vi "XYZ_translation_LastVersion.vi"() -> ()   [LabVIEW 2021]
uses:
  C:/Program Files (x86)/Control/SC3U.dll
  Program Files (x86)/Control/SC3U.dll
  <instrlib>/Xbox-One-Controller/Private/Type Defs/Indicators/Controller.ctl
  <instrlib>/Xbox-One-Controller/Private/Type Defs/Indicators/A.ctl
  <instrlib>/Xbox-One-Controller/Private/Type Defs/Indicators/B.ctl
  <instrlib>/Xbox-One-Controller/Private/Type Defs/Indicators/X.ctl
  <instrlib>/Xbox-One-Controller/Private/Type Defs/Indicators/Y.ctl
  <instrlib>/Xbox-One-Controller/Private/Type Defs/Indicators/Left Bumper.ctl
  <instrlib>/Xbox-One-Controller/Private/Type Defs/Indicators/Right Bumper.ctl
  <instrlib>/Xbox-One-Controller/Private/Type Defs/Indicators/View.ctl
  <instrlib>/Xbox-One-Controller/Private/Type Defs/Indicators/Menu.ctl
  <instrlib>/Xbox-One-Controller/Private/Type Defs/Indicators/Thumbstick_Analog.ctl
  <instrlib>/Xbox-One-Controller/Private/Type Defs/Indicators/Slider.ctl
  <instrlib>/Xbox-One-Controller/Private/Type Defs/Indicators/DPad.ctl
  <vilib>/Platform/TimedLoop/XDataNode/timing_clust.ctl
  <vilib>/Platform/TimedLoop/XDataNode/nitl_modes.ctl
  <vilib>/Platform/TimedLoop/XDataNode/wakeup.ctl
  <instrlib>/Xbox-One-Controller/Public/Open First Controller.vi
  <vilib>/Platform/TimedLoop/XDataNode/XDataNode.xnode
  <vilib>/Platform/TimedLoop/XDataNode/XDNodeRunTimeDep.lvlib
  <instrlib>/Xbox-One-Controller/LMH-Xbox-One-Controller.lvlib
panel:
  in  "Front Panel Window:Is Frontmost":bool
  in  "Displace Divided by 5":bool caption="Boolean 2"
  in  "Displace Multip by 5":bool caption="Boolean"
  out "Pos X":dbl
  out "Pos Z":dbl
  in  "Com Close 3":bool
  in  "Displace Z":i64=1
  out "Pos Y mm":dbl
  in  "Displace Y":i64
  in  "Com Close 2":bool
  in  "Stop Button":bool
  out "Controller":T1={"A Button"=FALSE, "B Button"=FALSE, "X Button"=FALSE, "Y Button"=FALSE, "Left Bumper"=FALSE, "Right Bumper"=FALSE, "View Button"=FALSE, "Menu Button"=FALSE, "Left Stick"={[], []}, "Right Stick"={[], []}, "Trigger"=0, "D-Pad"=5} {"Trigger" scale=32767.0..-32768.0}
  in  "SC3U":refnum<k24>(container)
  in  "Com Close":bool
  in  "Displace X":i64
  out "ConnectStatus":bool
  out "ComUsing":i16
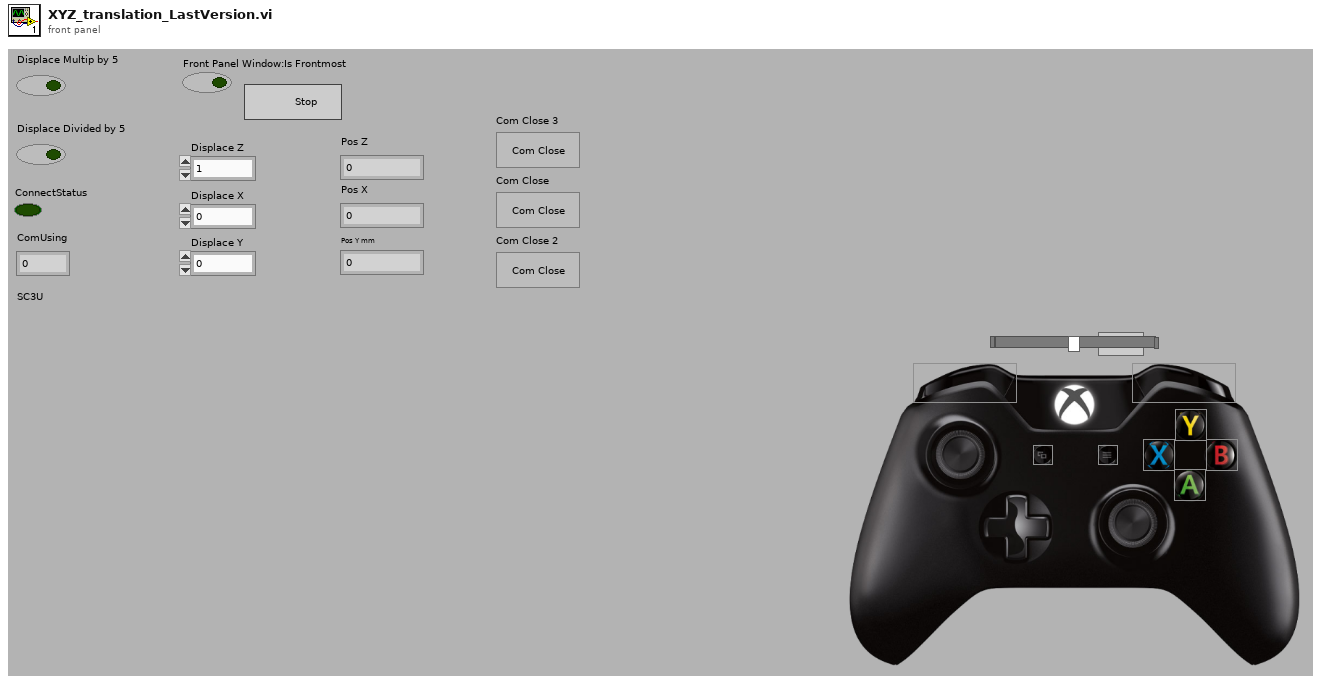
[diagram p1: front panel]
types:
  T1 = typedef "LMH-Xbox-One-Controller.lvlib/Controller.ctl" = cluster{"A Button":T2, "B Button":T3, "X Button":T4, "Y Button":T5, "Left Bumper":T6, "Right Bumper":T7, "View Button":T8, "Menu Button":T9, "Left Stick":T10, "Right Stick":T10, "Trigger":T11, "D-Pad":T12}
  T2 = typedef "LMH-Xbox-One-Controller.lvlib/A.ctl" = bool
  T3 = typedef "LMH-Xbox-One-Controller.lvlib/B.ctl" = bool
  T4 = typedef "LMH-Xbox-One-Controller.lvlib/X.ctl" = bool
  T5 = typedef "LMH-Xbox-One-Controller.lvlib/Y.ctl" = bool
  T6 = typedef "LMH-Xbox-One-Controller.lvlib/Left Bumper.ctl" = bool
  T7 = typedef "LMH-Xbox-One-Controller.lvlib/Right Bumper.ctl" = bool
  T8 = typedef "LMH-Xbox-One-Controller.lvlib/View.ctl" = bool
  T9 = typedef "LMH-Xbox-One-Controller.lvlib/Menu.ctl" = bool
  T10 = typedef "LMH-Xbox-One-Controller.lvlib/Thumbstick_Analog.ctl" = cluster{i32[], i32[]}
  T11 = typedef "LMH-Xbox-One-Controller.lvlib/Slider.ctl" = i32
  T12 = typedef "LMH-Xbox-One-Controller.lvlib/DPad.ctl" = u16
  T13 = typedef "XDNodeRunTimeDep.lvlib/timing_clust.ctl" = cluster{"Expected End [f-1]":u64, "Actual End [f-1]":u64, "Finished Late? [f-1]":bool, "Expected End [i-1]":u64, "Actual End [i-1]":u64, "Finished Late? [i-1]":bool, "Expected Start [i]":u64, "Actual Start [i]":u64, "Expected Start [f]":u64, "Actual Start [f]":u64, "Source Name":string, "Structure Name":string, "Period":i64, "Deadline":i64, "Offset":i64, "Start":i64, "Priority":i32, "Timeout":i32, "Mode":T14, "Wakeup Reason":T15, "Error":errorcluster, "Source Type":string, "Secondary Source Type":string, "Global End Time":u64, "Global Start Time":u64, "Frame Duration":u64, "Iteration Duration":u64, "Assigned CPU":i32, "I/O Scan Engine Mode":u32}
  T14 = typedef "XDNodeRunTimeDep.lvlib/nitl_modes.ctl" = enum32{"No Change", "Process missed periods, maintain original phase", "Discard missed periods, maintain original phase", "Process missed periods, ignore original phase", "Discard missed periods, ignore original phase"}
  T15 = typedef "XDNodeRunTimeDep.lvlib/wakeup.ctl" = enum32{"Normal", "Aborted", "Asynchronous wakeup", "Timing source error", "Timed loop error", "Timeout"}
  T16 = typedef "LMH-Xbox-One-Controller.lvlib/Xbox One Controller Ref.ctl" = cluster{"Controller Ref":refnum<k1>, "Event Refnum":refnum<event-registration>, "Worker Ref":refnum<vi>}
  T17 = typedef "LMH-Xbox-One-Controller.lvlib/All Axis Data.ctl" = cluster{"Left Stick":cluster{"X Axis":i32, "Y Axis":i32}, "Right Stick":cluster{"X Axis":i32, "Y Axis":i32}, "Triggers":i32, "D-Pad":T18}
  T18 = typedef "LMH-Xbox-One-Controller.lvlib/DPad Enum.ctl" = enum16{"Idle", "Up", "Up / Right", "Right", "Down / Right", "Down", "Down / Left", "Left", "Up / Left"}
  T19 = typedef "LMH-Xbox-One-Controller.lvlib/All Buttons Visual.ctl" = cluster{"A":T2, "B":T3, "X":T4, "Y":T5, "Left Bumper":T6, "Right Bumper":T7, "View Button":T8, "Menu Button":T9, "Left Stick":T20, "Right Stick":T20}
  T20 = typedef "LMH-Xbox-One-Controller.lvlib/Thumbstick.ctl" = bool
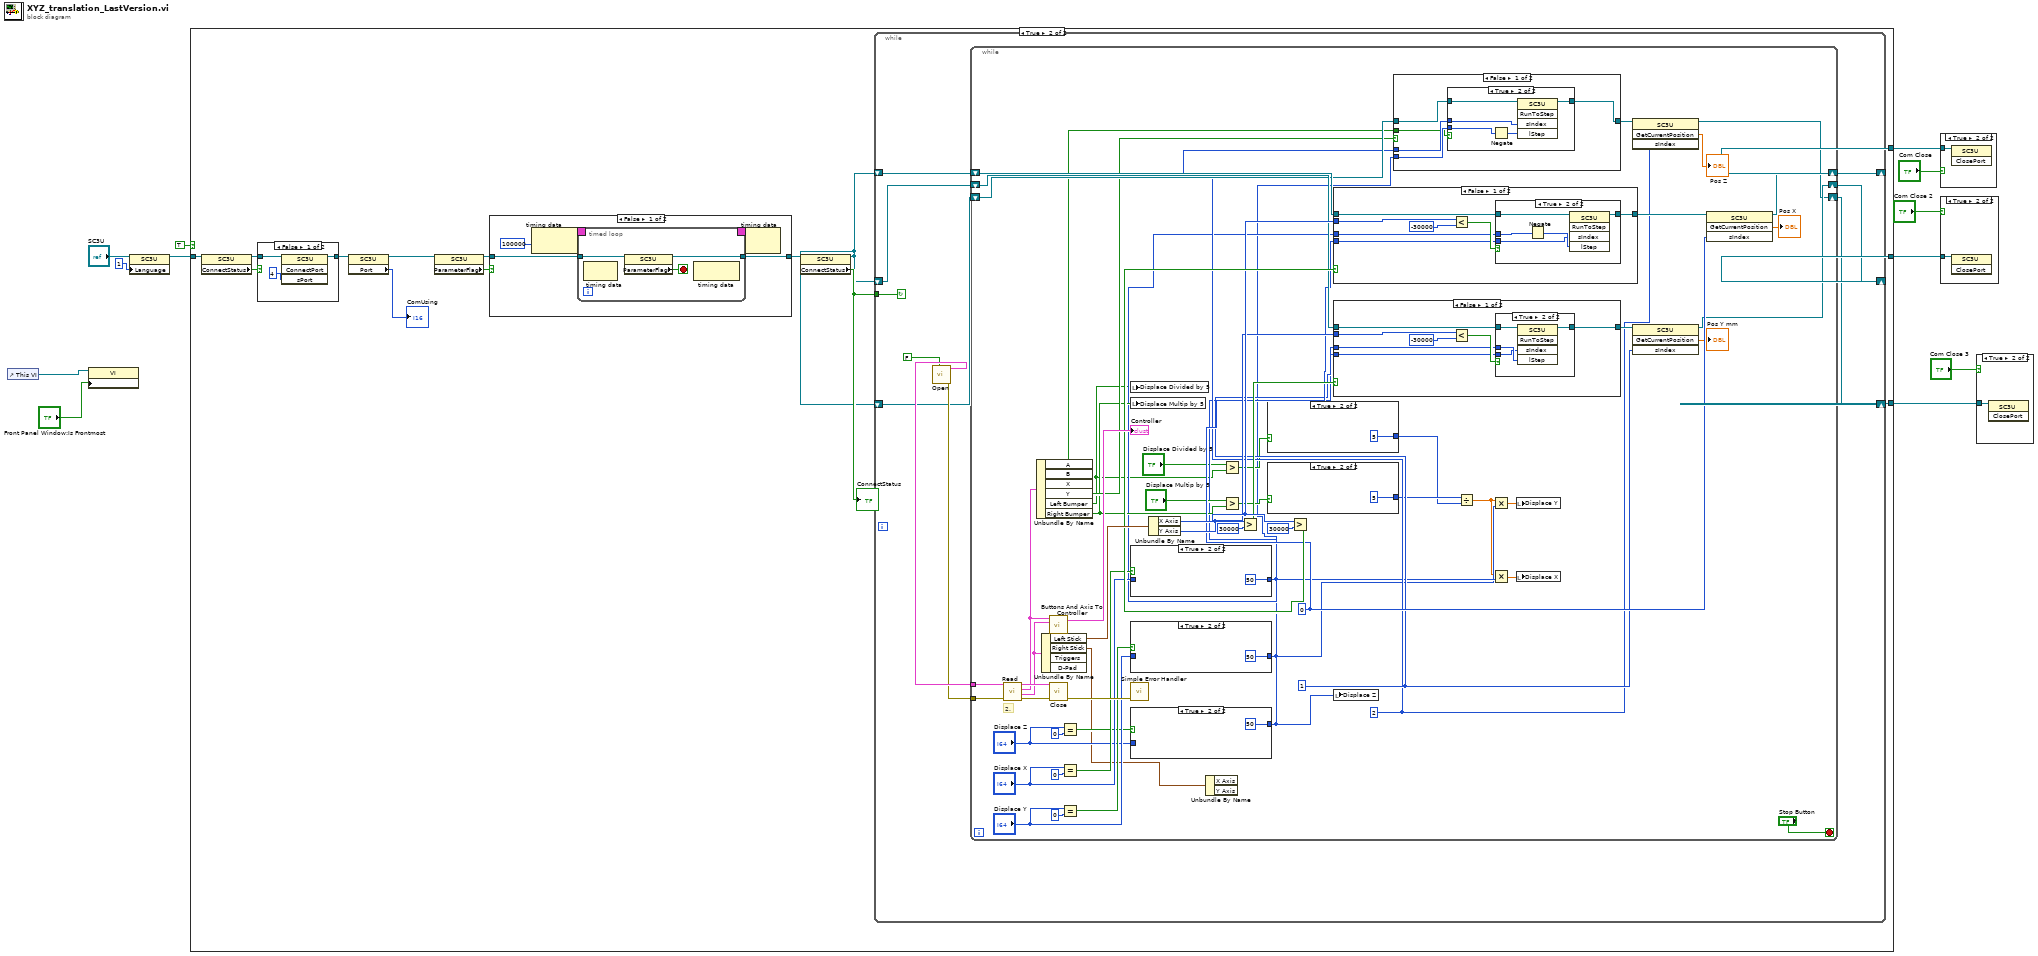
[diagram p0: block diagram]
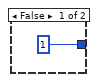
[diagram p7: hidden frame]
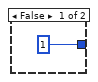
[diagram p9: hidden frame]
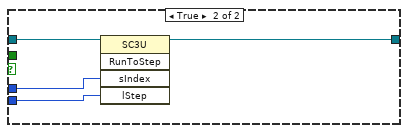
[diagram p12: hidden frame]
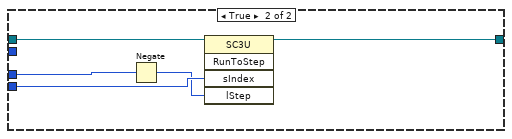
[diagram p14: hidden frame]
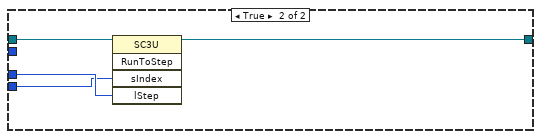
[diagram p16: hidden frame]
diagram:
  n1 = control-ref of="This VI"() -> (w2:refnum<vi>)
  n2 = property class="VI"(reference=w2, "Front Panel.IsFrontmost"="Front Panel Window:Is Frontmost") -> ()  [unwired: 1 in, 2 out]
  n3 = property class="SC3U"(reference="SC3U", "Language"=i16 1 ("intLanguage")) -> (reference out=w5:refnum<k24>)  [unwired: 1 in, 1 out]
  n4 = case shown="True" TRUE {
    tunnel: [_ w16] -> w8
    tunnel: w5 -> [_ w25]
    tunnel: [_ w15] -> w6
    tunnel: [_ w13] -> w3
    frame False {
    }
    frame True {
      n5 = property class="SC3U"(reference=w25) -> (reference out=w24:refnum<k24>, "ConnectStatus"=w23:bool)  [unwired: 1 in, 1 out]
      n6 = case shown="False" w23 {
        tunnel: w24 -> [w170 w171]
        tunnel: [w169 w171] -> w22
        frame False {
          n7 = invoke class="SC3U" method="ConnectPort"(reference=w170, "sPort"=i16 4 ("ComUsing")) -> (reference out=w169:refnum<k24>)  [unwired: 2 in, 3 out]
        }
        frame True {
        }
      }
      n8 = property class="SC3U"(reference=w22) -> (reference out=w20:refnum<k24>, "Port"=→"ComUsing":i16)  [unwired: 1 in, 1 out]
      n9 = property class="SC3U"(reference=w20) -> (reference out=w19:refnum<k24>, "ParameterFlag"=w18:bool)  [unwired: 1 in, 1 out]
      n10 = case shown="False" w18 {
        tunnel: w19 -> [w154 w167]
        tunnel: [w153 w167] -> w26
        frame False {
          n11 = node-c288(i64 100000 ("周期")) -> (w157:T13)
          n12 = timed-loop {
            timing: w157 -> [_]
            timing-out: [_] -> w156
            tunnel: w154 -> [w160]
            tunnel: [w159] -> w153
            stop <- w158 stop-if-true
            n13 = node-c288() -> ()  [unwired: 1 in, 1 out]
            n14 = property class="SC3U"(reference=w160) -> (reference out=w159:refnum<k24>, "ParameterFlag"=w158:bool)  [unwired: 1 in, 1 out]
            n15 = node-c288() -> ()  [unwired: 1 in, 1 out]
          }
          n16 = node-c288(w156) -> ()  [unwired: 1 out]
        }
        frame True {
        }
      }
      n17 = property class="SC3U"(reference=w26) -> (reference out=w14:refnum<k24>, "ConnectStatus"=w17:bool)  [unwired: 1 in, 1 out]
      "ConnectStatus" <- w17
      n18 = while {
        shift-right: [w36] -> w16
        shift-left: w14 -> [w35]
        tunnel: w17 -> [w34]
        shift-right: [w29] -> w15
        shift-left: w14 -> [w30]
        shift-right: [w27] -> w13
        shift-left: w14 -> [w28]
        stop <- w34 continue-if-true
        n19 = call-poly <instrlib>:"Open.vi"("Enable Events (T)"=FALSE) -> ("Error Out"=w32:errorcluster, "Xbox One Controller"=w33:T16)  [unwired: 8 in, 1 out]
        n20 = while {
          tunnel: w33 -> [w90]
          tunnel: w32 -> [w89]
          shift-right: [w76] -> w36
          shift-left: w35 -> [w93]
          shift-right: [w73] -> w29
          shift-left: w30 -> [w79]
          shift-right: [w67] -> w27
          shift-left: w28 -> [w68]
          stop <- "Stop Button" stop-if-true
          w66 = 2
          w71 = 1
          w75 = 0
          # "2."
          n21 = call <instrlib>:"Read.vi"("Error In"=w89, "Xbox One Controller Ref"=w90) -> ("Error Out"=w87:errorcluster, "All Axis"=w85:T17, "Buttons"=w64:T19, "Xbox One Controller Ref"=w86:T16)  [unwired: 6 in]
          n22 = Unbundle By Name(w64) -> ("A"=w63:T2, "Y"=w62:T5, "Left Bumper"=w46:T6, "Right Bumper"=w57:T7)  [unwired: 2 out]
          n23 = Unbundle By Name(w85) -> ("Left Stick"=w92:cluster{"X Axis":i32, "Y Axis":i32}, "Right Stick"=w37:cluster{"X Axis":i32, "Y Axis":i32})  [unwired: 2 out]
          n24 = call <instrlib>:"Buttons And Axis To Controller.vi"("All Axis"=w85, "Buttons"=w64) -> ("Controller"=→"Controller":T1)  [unwired: 5 in]
          n25 = call <instrlib>:"Close.vi"("Error In"=w87, "Xbox One Controller Ref"=w86) -> ("Error Out"=w88:errorcluster)  [unwired: 9 in]
          n26 = Equal?(x="Displace Z", y=0) -> (x = y?=w41:bool)
          n27 = Equal?(x="Displace X", y=0) -> (x = y?=w60:bool)
          n28 = Equal?(x="Displace Y", y=0) -> (x = y?=w50:bool)
          n29 = local write "Displace Divided by 5"(w46) -> ()
          n30 = local write "Displace Multip by 5"(w57) -> ()
          n31 = case shown="True" w60 {
            tunnel: [w102 50] -> w54
            tunnel: "Displace X" -> [w102 _]
            frame False {
            }
            frame True {
            }
          }
          n32 = case shown="True" w50 {
            tunnel: [w98 50] -> w48
            tunnel: "Displace Y" -> [w98 _]
            frame False {
            }
            frame True {
            }
          }
          n33 = call <vilib>:"Simple Error Handler.vi"("error in (no error)"=w88) -> ()  [unwired: 4 in, 5 out]
          n34 = case shown="True" w41 {
            tunnel: [w94 50] -> w38
            tunnel: "Displace Z" -> [w94 _]
            frame False {
            }
            frame True {
            }
          }
          n35 = Unbundle By Name(w92) -> ("X Axis"=w82:i32, "Y Axis"=w78:i32)
          n36 = Unbundle By Name(w37) -> ()  [unwired: 2 out]
          n37 = Greater?(x="Displace Divided by 5", y=w46) -> (0:w45:T6)
          n38 = Greater?(x="Displace Multip by 5", y=w57) -> (0:w55:T7)
          n39 = Greater?(x=w78, y=30000) -> (0:w80:bool)
          n40 = case shown="True" w45 {
            tunnel: [1 5] -> w43
            frame False {
            }
            frame True {
            }
          }
          n41 = case shown="True" w55 {
            tunnel: [1 5] -> w44
            frame False {
            }
            frame True {
            }
          }
          n42 = Greater?(x=w82, y=30000) -> (0:w83:bool)
          n43 = case shown="False" w83 {
            tunnel: [w141 w149] -> w77
            tunnel: w93 -> [w142 w152]
            tunnel: w82 -> [w140 _]
            tunnel: w54 -> [w137 w151]
            tunnel: w75 -> [w136 w150]
            frame False {
              n44 = Less?(x=w140, y=-30000) -> (x < y?=w138:bool)
              n45 = case shown="True" w138 {
                tunnel: w142 -> [w143 w148]
                tunnel: [w143 w144] -> w141
                tunnel: w137 -> [_ w146]
                tunnel: w136 -> [_ w145]
                frame False {
                }
                frame True {
                  n46 = Negate(x=w146) -> (-x=w147:i64)
                  n47 = invoke class="SC3U" method="RunToStep"(reference=w148, "sIndex"=w145, "lStep"=w147) -> (reference out=w144:refnum<k24>)  [unwired: 2 in, 4 out]
                }
              }
            }
            frame True {
              n48 = invoke class="SC3U" method="RunToStep"(reference=w152, "sIndex"=w150, "lStep"=w151) -> (reference out=w149:refnum<k24>)  [unwired: 2 in, 4 out]
            }
          }
          n49 = case shown="False" w80 {
            tunnel: [w124 w133] -> w74
            tunnel: w79 -> [w125 w135]
            tunnel: w78 -> [w123 _]
            tunnel: w48 -> [w119 w132]
            tunnel: w71 -> [w120 w134]
            frame False {
              n50 = Less?(x=w123, y=-30000) -> (x < y?=w121:bool)
              n51 = case shown="True" w121 {
                tunnel: w125 -> [w126 w130]
                tunnel: [w126 w127] -> w124
                tunnel: w119 -> [_ w129]
                tunnel: w120 -> [_ w128]
                frame False {
                }
                frame True {
                  n52 = invoke class="SC3U" method="RunToStep"(reference=w130, "sIndex"=w128, "lStep"=w129) -> (reference out=w127:refnum<k24>)  [unwired: 2 in, 4 out]
                }
              }
            }
            frame True {
              n53 = Negate(x=w132) -> (-x=w131:i64)
              n54 = invoke class="SC3U" method="RunToStep"(reference=w135, "sIndex"=w134, "lStep"=w131) -> (reference out=w133:refnum<k24>)  [unwired: 2 in, 4 out]
            }
          }
          n55 = local write "Displace Z"(w38) -> ()
          n56 = case shown="False" w62 {
            tunnel: w66 -> [w106 w118]
            tunnel: w38 -> [w105 w117]
            tunnel: w68 -> [w108 w116]
            tunnel: [w107 w115] -> w70
            tunnel: w63 -> [w104 _]
            frame False {
              n57 = case shown="True" w104 {
                tunnel: w108 -> [w109 w114]
                tunnel: [w109 w113] -> w107
                tunnel: w106 -> [_ w112]
                tunnel: w105 -> [_ w110]
                frame False {
                }
                frame True {
                  n58 = Negate(x=w110) -> (-x=w111:i64)
                  n59 = invoke class="SC3U" method="RunToStep"(reference=w114, "sIndex"=w112, "lStep"=w111) -> (reference out=w113:refnum<k24>)  [unwired: 2 in, 4 out]
                }
              }
            }
            frame True {
              n60 = invoke class="SC3U" method="RunToStep"(reference=w116, "sIndex"=w118, "lStep"=w117) -> (reference out=w115:refnum<k24>)  [unwired: 2 in, 4 out]
            }
          }
          n61 = Divide(x=w44, y=w43) -> (x/y=w39:dbl)
          n62 = Multiply(x=w39, y=w48) -> (x*y=w49:dbl)
          n63 = Multiply(x=w39, y=w54) -> (x*y=w53:dbl)
          n64 = local write "Displace Y"(w49) -> ()
          n65 = local write "Displace X"(w53) -> ()
          n66 = invoke class="SC3U" method="GetCurrentPosition"(reference=w70, "sIndex"=w66) -> (reference out=w67:refnum<k24>, "GetCurrentPosition"=→"Pos Z":dbl)  [unwired: 2 in, 2 out]
          n67 = invoke class="SC3U" method="GetCurrentPosition"(reference=w74, "sIndex"=w71) -> (reference out=w73:refnum<k24>, "GetCurrentPosition"=→"Pos Y mm":dbl)  [unwired: 2 in, 2 out]
          n68 = invoke class="SC3U" method="GetCurrentPosition"(reference=w77, "sIndex"=w75) -> (reference out=w76:refnum<k24>, "GetCurrentPosition"=→"Pos X":dbl)  [unwired: 2 in, 2 out]
        }
      }
    }
  }
  n69 = case shown="True" "Com Close" {
    tunnel: w8 -> [_ w172]
    frame False {
    }
    frame True {
      n70 = invoke class="SC3U" method="ClosePort"(reference=w172) -> ()  [unwired: 2 in, 3 out]
    }
  }
  n71 = case shown="True" "Com Close 2" {
    tunnel: w6 -> [_ w173]
    frame False {
    }
    frame True {
      n72 = invoke class="SC3U" method="ClosePort"(reference=w173) -> ()  [unwired: 2 in, 3 out]
    }
  }
  n73 = case shown="True" "Com Close 3" {
    tunnel: w3 -> [_ w174]
    frame False {
    }
    frame True {
      n74 = invoke class="SC3U" method="ClosePort"(reference=w174) -> ()  [unwired: 2 in, 3 out]
    }
  }
